vi "BRig_dataExp_FreeReward_Count2.vi"() -> (2 "output_FreeReward_Count":i32)   [LabVIEW 2014]
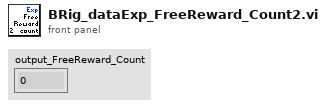
[diagram p1: front panel]
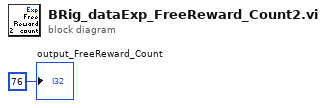
[diagram p0: block diagram]
diagram:
  "output_FreeReward_Count" <- 76 ("output_iBlock")
